vi "12.4 MorphReconstruct-Gray.vi"() -> ()   [LabVIEW 2016]
doc: "This example shows how to use the Edge Tool in NI Vision. The Edge Tool finds edges (or sharp transitions in the pixels values) along a given line or ROI profile. The Edge Tool is a precursor function to many of the gauging and inspection tasks. For example, the location of the edges found along a line profile across an object can interpreted as the boundaries of the object whose dimensions have to be measured for a gauging application or the presence of a crack in the surface of an object for an inspection application."
uses:
  <vilib>/vision/NI_Vision_Development_Module.lvlib
panel:
  in  "Operation":enum16{"Dilate", "Erode"}(ring)
  out "Src":T1(plugin-control)
  out "Dst":T1(plugin-control)
  in  "Stop":bool
  # "Instruction:\n1. Run the VI;\n2. Draw ROI in left \nImgage;\n3. Select different\noperation to see the\nresults in right."
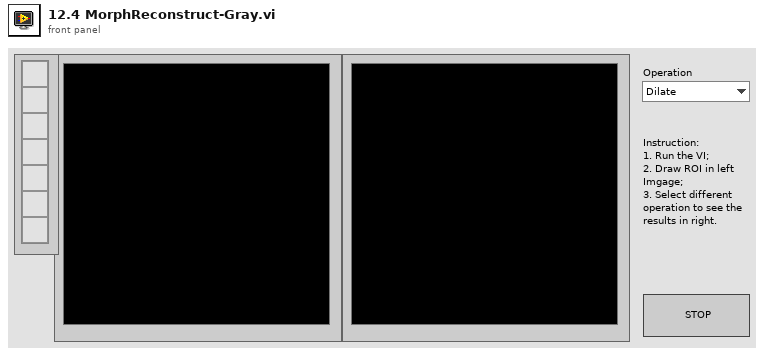
[diagram p1: front panel]
types:
  T1 = typedef "IMAQ Image.ctl" = refnum<image>
  T2 = typedef "Image Type" = u32
  T3 = cluster{"Global Rectangle":i32[], "Contours":cluster{"Contour Type":u32, "ROI Type":u32, "Points":i32[]}[]}
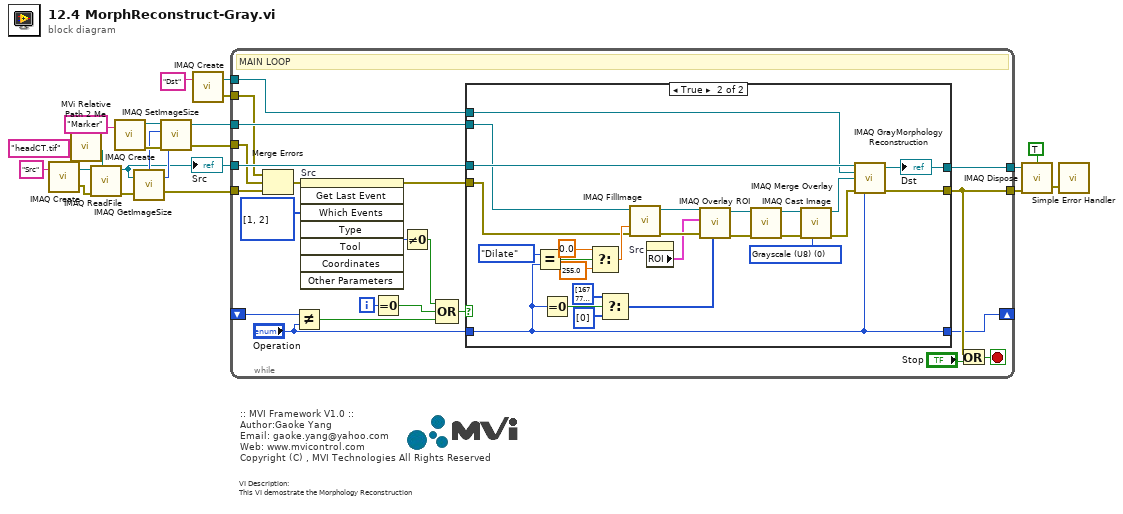
[diagram p0: block diagram]
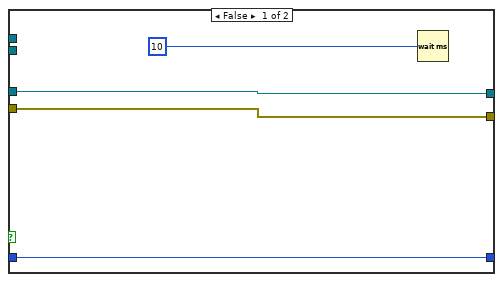
[diagram p2: hidden frame]
diagram:
  # "VI Description:\nThis VI demostrate the Morphology Reconstruction"
  # ":: MVI Framework V1.0 ::\nAuthor:Gaoke Yang\nEmail: gaoke.yang@yahoo.com\nWeb: www.mvicontrol.com\nCopyright (C) , MVI Technologies All Rights Reserved"
  n1 = call "IMAQ Create"("Image Name"="Src") -> ("New Image"=w21:T1, "error out"=w20:errorcluster)  [unwired: 4 in]
  n2 = call "MVi Relative Path 2 Me.vi"("Relative Path"="headCT.tif" ("name or relative path")) -> ("Appended Dir"=w16:path)  [unwired: 5 in, 1 out]
  n3 = call "IMAQ ReadFile"("File Path"=w16, "error in (no error)"=w20, "Image"=w21) -> ("error out"=w9:errorcluster, "Image Out"=w3:T1)  [unwired: 4 in, 3 out]
  "Src" <- w3
  n4 = call "IMAQ Create"("Image Name"="Marker") -> ("New Image"=w7:T1, "error out"=w8:errorcluster)  [unwired: 4 in]
  n5 = call "IMAQ GetImageSize"("Image"=w3, "error in (no error)"=w9) -> ("Y Resolution"=w6:i32, "X Resolution"=w5:i32, "error out"=w4:errorcluster)  [unwired: 2 out]
  n6 = call "IMAQ SetImageSize"("error in (no error)"=w8, "Y Resolution"=w6, "X Resolution"=w5, "Image"=w7) -> ("error out"=w2:errorcluster, "Image Out"=w1:T1)  [unwired: 1 in]
  n7 = call "IMAQ Create"("Image Name"="Dst") -> ("New Image"=w11:T1, "error out"=w10:errorcluster)  [unwired: 4 in]
  n8 = while "MAIN LOOP" {
    tunnel: w3 -> [w44]
    tunnel: w4 -> [w28]
    tunnel: [w40] -> w19
    tunnel: [w41] -> w18
    shift-right: [w37] -> _
    shift-left: _ -> [w35]
    tunnel: w1 -> [w33]
    tunnel: w2 -> [w26]
    tunnel: w11 -> [w24]
    tunnel: w10 -> [w25]
    i -> [w39]
    stop <- w42 stop-if-true
    w31 = i32[] [1, 2] items=["No Event"=0, "Click Event"=1, "Draw Event"=2, "Size Event"=4, "Scroll Event"=5, "Double Click Event"=8] ("Which Events")
    # "MAIN LOOP"
    n9 = Merge Errors(w25, w26, w28) -> (w27:errorcluster)
    n10 = Not Equal?(x=w35, y="Operation") -> (x != y?=w34:bool)
    n11 = invoke on="Src" class="ImageControl" method="Get Last Event"(error in=w27, "Which Events"=w31) -> (error out=w32:errorcluster, "Type"=w30:i32)  [unwired: 6 in, 6 out]
    n12 = Equal To 0?(x=w39) -> (x = 0?=w36:bool)
    n13 = Not Equal To 0?(x=w30) -> (x != 0?=w29:bool)
    n14 = Compound Arithmetic op=OR(w29, w36, w34) -> (w38:bool)
    n15 = case shown="True" w38 {
      tunnel: w32 -> [w47 w69]
      tunnel: w44 -> [w48 w55]
      tunnel: [w48 w56] -> w41
      tunnel: [w47 w57] -> w40
      tunnel: [w45 w51] -> w37
      tunnel: "Operation" -> [w45 w51]
      tunnel: w33 -> [_ w54]
      tunnel: w24 -> [_ w53]
      frame False {
        n16 = Wait (ms)(milliseconds to wait=u32 10) -> ()  [unwired: 1 out]
      }
      frame True {
        w62 = T2 0 items=["Grayscale (U8)", "Grayscale (I16)", "Grayscale (SGL)", "Complex (CSG)", "RGB (U32)", "HSL (U32)", "RGB (U64)", "Grayscale (U16)"] ("Image Type")
        n17 = Equal?(x=enum16{"Dilate", "Erode"}."Dilate" ("Operation"), y=w51) -> (x = y?=w74:bool)
        n18 = Equal To 0?(x=w51) -> (x = 0?=w63:bool)
        n19 = Select(t=sgl 0.0 ("Pixel Value (U8, U16, I16, Float)"), s=w74, f=sgl 255.0 ("Pixel Value (U8, U16, I16, Float)")) -> (s? t:f=w71:sgl)
        n20 = Select(t=u32[] [16777215] ("Colors (Green)"), s=w63, f=u32[] [0] ("Colors (Green)")) -> (s? t:f=w66:u32[])
        n21 = call "IMAQ FillImage"("error in (no error)"=w69, "Pixel Value (U8, U16, I16, Float)"=w71, "Image"=w54) -> ("error out"=w60:errorcluster, "Image Out"=w61:T1)  [unwired: 4 in, 3 out]
        n22 = property on="Src" class="ImageControl"() -> ("ROI"=w59:T3)  [unwired: 2 in, 2 out]
        n23 = call "IMAQ Overlay ROI"("Colors (Green)"=w66, "error in (no error)"=w60, "ROI Descriptor"=w59, "Image"=w61) -> ("error out"=w67:errorcluster, "Image Out"=w50:T1)  [unwired: 2 in, 4 out]
        n24 = call "IMAQ Merge Overlay"("error in (no error)"=w67, "Image Src"=w50) -> ("error out"=w68:errorcluster, "Image Dst Out"=w49:T1)  [unwired: 3 in, 5 out]
        n25 = call "IMAQ Cast Image"("Image Type"=w62, "error in (no error)"=w68, "Image Src"=w49) -> ("error out"=w58:errorcluster, "Image Dst Out"=w52:T1)  [unwired: 3 in, 4 out]
        n26 = call "IMAQ GrayMorphology Reconstruction"("Image Src"=w55, "Image Dst"=w53, "Image Marker"=w52, "error in (no error)"=w58, "Operation"=w51) -> ("Image Dst Out"=w56:T1, "error out"=w57:errorcluster)  [unwired: 9 in]
        "Dst" <- w56
      }
    }
    n27 = Or(x=w40, y="Stop") -> (x .or. y?=w42:bool)
  }
  n28 = call "IMAQ Dispose"("All Images? (No)"=TRUE, "Image"=w18, "error in (no error)"=w19) -> ("error out"=w15:errorcluster)  [unwired: 3 in]
  n29 = call <vilib>:"Simple Error Handler.vi"("error in (no error)"=w15) -> ()  [unwired: 4 in, 5 out]
